vi "CRIO_main.vi"() -> ()   [LabVIEW 2019]
uses:
  <vilib>/Platform/TimedLoop/XDataNode/timing_clust.ctl
  <vilib>/Platform/TimedLoop/XDataNode/nitl_modes.ctl
  <vilib>/Platform/TimedLoop/XDataNode/wakeup.ctl
  <vilib>/DAQmx/read.llb/DAQmx Read (Analog DBL 1Chan 1Samp).vi
  <vilib>/DAQmx/create/channels.llb/DAQmx Create Channel (AI-Voltage-Basic).vi
  <vilib>/DAQmx/configure/timing.llb/DAQmx Timing (Sample Clock).vi
  <vilib>/DAQmx/miscellaneous.llb/DAQmx Fill In Error Info.vi
  <vilib>/platform/TimedLoop/XDataNode/XDataNode.xnode
  <vilib>/Platform/TimedLoop/XDataNode/XDNodeRunTimeDep.lvlib
  <resource>/objmgr/ni.dex.rc
panel:
  out "error out 7":errorcluster
  out "error out 6":errorcluster
  out "Boolean":bool
  out "error out 5":errorcluster
  out "error out 4":errorcluster
  out "error out 3":errorcluster
  out "error out 2":errorcluster
  out "error out":errorcluster
  in  "stop":bool
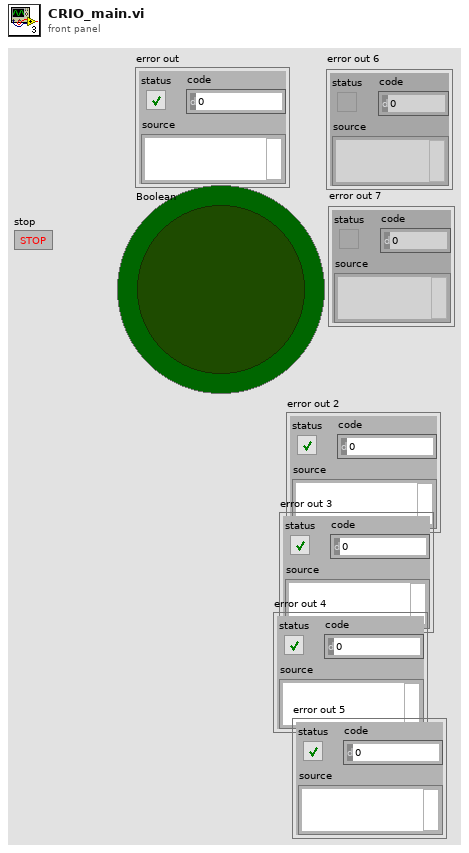
[diagram p1: front panel]
types:
  T1 = typedef "XDNodeRunTimeDep.lvlib/timing_clust.ctl" = cluster{"Expected End [f-1]":u64, "Actual End [f-1]":u64, "Finished Late? [f-1]":bool, "Expected End [i-1]":u64, "Actual End [i-1]":u64, "Finished Late? [i-1]":bool, "Expected Start [i]":u64, "Actual Start [i]":u64, "Expected Start [f]":u64, "Actual Start [f]":u64, "Source Name":string, "Structure Name":string, "Period":i64, "Deadline":i64, "Offset":i64, "Start":i64, "Priority":i32, "Timeout":i32, "Mode":T2, "Wakeup Reason":T3, "Error":errorcluster, "Source Type":string, "Secondary Source Type":string, "Global End Time":u64, "Global Start Time":u64, "Frame Duration":u64, "Iteration Duration":u64, "Assigned CPU":i32, "I/O Scan Engine Mode":u32}
  T2 = typedef "XDNodeRunTimeDep.lvlib/nitl_modes.ctl" = enum32{"No Change", "Process missed periods, maintain original phase", "Discard missed periods, maintain original phase", "Process missed periods, ignore original phase", "Discard missed periods, ignore original phase"}
  T3 = typedef "XDNodeRunTimeDep.lvlib/wakeup.ctl" = enum32{"Normal", "Aborted", "Asynchronous wakeup", "Timing source error", "Timed loop error", "Timeout"}
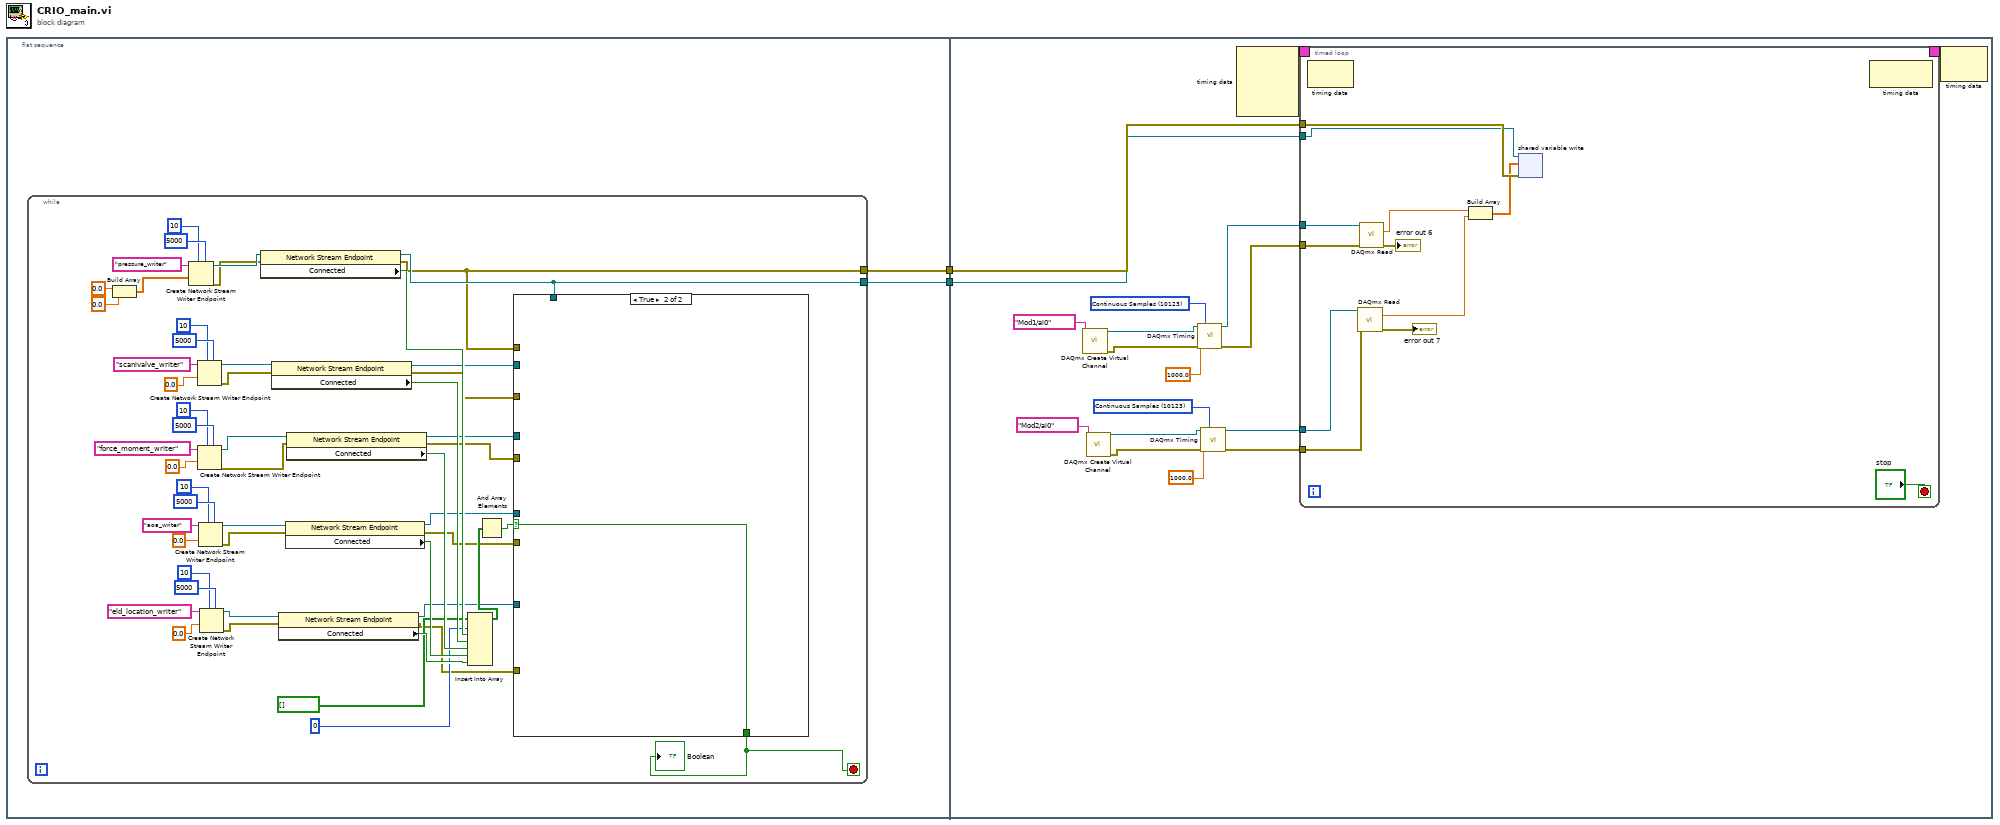
[diagram p0: block diagram]
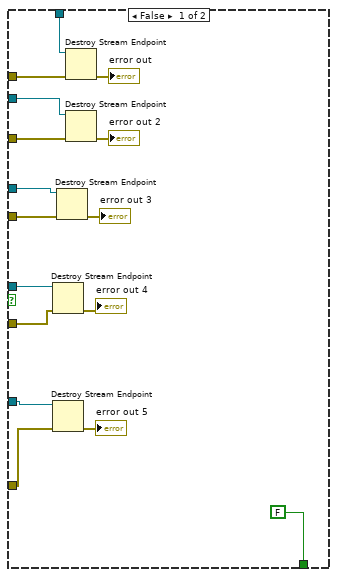
[diagram p2: hidden frame]
diagram:
  n1 = flat-sequence {
    tunnel: [w4] -> w2
    tunnel: [w3] -> w1
    tunnel: w2 -> [w89]
    tunnel: w1 -> [w88]
    frame #0 {
      n2 = while {
        tunnel: [w15] -> w4
        tunnel: [w16] -> w3
        stop <- w8 stop-if-true
        n3 = Build Array(0.0 ("element"), 0.0 ("element")) -> (w5:dbl[])
        n4 = Create Network Stream Writer Endpoint(5:5000 ("timeout in ms (-1)"), 7:10 ("writer buffer size"), 9:w5, 11:"pressure_writer" ("writer name")) -> (0:w36:errorcluster, 3:w37:refnum<k21>)  [unwired: 3 in]
        n5 = Create Network Stream Writer Endpoint(5:5000 ("timeout in ms (-1)"), 7:10 ("writer buffer size"), 9:0.0, 11:"scanivalve_writer" ("writer name")) -> (0:w31:errorcluster, 3:w32:refnum<k21>)  [unwired: 3 in]
        n6 = Create Network Stream Writer Endpoint(5:5000 ("timeout in ms (-1)"), 7:10 ("writer buffer size"), 9:0.0, 11:"force_moment_writer" ("writer name")) -> (0:w29:errorcluster, 3:w30:refnum<k21>)  [unwired: 3 in]
        n7 = Create Network Stream Writer Endpoint(5:5000 ("timeout in ms (-1)"), 7:10 ("writer buffer size"), 9:0.0, 11:"aoa_writer" ("writer name")) -> (0:w25:errorcluster, 3:w26:refnum<k21>)  [unwired: 3 in]
        n8 = Create Network Stream Writer Endpoint(5:5000 ("timeout in ms (-1)"), 7:10 ("writer buffer size"), 9:0.0, 11:"eld_location_writer" ("writer name")) -> (0:w22:errorcluster, 3:w23:refnum<k21>)  [unwired: 3 in]
        n9 = property class="Network Stream Endpoint"(reference=w37, error in=w36) -> (reference out=w16:refnum<k21>, error out=w15:errorcluster, "Connected"=w35:bool)
        n10 = property class="Network Stream Endpoint"(reference=w32, error in=w31) -> (reference out=w18:refnum<k21>, error out=w17:errorcluster, "Connected"=w28:bool)
        n11 = property class="Network Stream Endpoint"(reference=w23, error in=w22) -> (reference out=w10:refnum<k21>, error out=w9:errorcluster, "Connected"=w21:bool)
        n12 = property class="Network Stream Endpoint"(reference=w26, error in=w25) -> (reference out=w12:refnum<k21>, error out=w11:errorcluster, "Connected"=w24:bool)
        n13 = property class="Network Stream Endpoint"(reference=w30, error in=w29) -> (reference out=w14:refnum<k21>, error out=w13:errorcluster, "Connected"=w27:bool)
        n14 = Insert Into Array(array=bool[] [], index=0, new element #1=w35, new element #2=w28, new element #3=w27, new element #4=w24, new element #5=w21) -> (w34:bool[])
        n15 = And Array Elements(Boolean array=w34) -> (logical AND=w33:bool)
        n16 = case shown="True" w33 {
          selector: w33 -> [_ w73]
          tunnel: w18 -> [w67 _]
          tunnel: w17 -> [w66 _]
          tunnel: w16 -> [w65 _]
          tunnel: w15 -> [w64 _]
          tunnel: w14 -> [w63 _]
          tunnel: w13 -> [w62 _]
          tunnel: w12 -> [w61 _]
          tunnel: w11 -> [w60 _]
          tunnel: w10 -> [w59 _]
          tunnel: w9 -> [w58 _]
          tunnel: [FALSE w73] -> w8
          frame False {
            n17 = Destroy Stream Endpoint(8:w60, 11:w61) -> (0:→"error out 4":errorcluster)
            n18 = Destroy Stream Endpoint(8:w58, 11:w59) -> (0:→"error out 5":errorcluster)
            n19 = Destroy Stream Endpoint(8:w62, 11:w63) -> (0:→"error out 3":errorcluster)
            n20 = Destroy Stream Endpoint(8:w64, 11:w65) -> (0:→"error out":errorcluster)
            n21 = Destroy Stream Endpoint(8:w66, 11:w67) -> (0:→"error out 2":errorcluster)
          }
          frame True {
          }
        }
        "Boolean" <- w8
      }
    }
    frame #1 {
      w79 = 10123 items=["Finite Samples"=10178, "Continuous Samples"=10123, "Hardware Timed Single Point"=12522] ("sample mode")
      w86 = 10123 items=["Finite Samples"=10178, "Continuous Samples"=10123, "Hardware Timed Single Point"=12522] ("sample mode")
      n22 = call-poly <vilib>:"DAQmx Create Virtual Channel.vi"("physical channels"=tag "Mod1/ai0") -> ("task out"=w83:refnum<k21>, "error out"=w82:errorcluster)  [unwired: 13 in]
      n23 = call-poly <vilib>:"DAQmx Create Virtual Channel.vi"("physical channels"=tag "Mod2/ai0") -> ("task out"=w77:refnum<k21>, "error out"=w76:errorcluster)  [unwired: 13 in]
      n24 = call-poly <vilib>:"DAQmx Timing.vi"("task/channels in"=w83, "sample mode"=w86, "rate"=1000.0, "error in"=w82) -> ("task out"=w84:refnum<k21>, "error out"=w81:errorcluster)  [unwired: 10 in]
      n25 = call-poly <vilib>:"DAQmx Timing.vi"("task/channels in"=w77, "sample mode"=w79, "rate"=1000.0, "error in"=w76) -> ("task out"=w75:refnum<k21>, "error out"=w74:errorcluster)  [unwired: 10 in]
      n26 = node-c288() -> (w91:T1)  [unwired: 4 in]
      n27 = timed-loop {
        timing: w91 -> [_]
        timing-out: [_] -> w90
        tunnel: w89 -> [w103]
        tunnel: w88 -> [w102]
        tunnel: w84 -> [w100]
        tunnel: w81 -> [w99]
        tunnel: w75 -> [w96]
        tunnel: w74 -> [w95]
        stop <- "stop" stop-if-true
        n28 = node-c288() -> ()  [unwired: 1 in, 1 out]
        n29 = call-poly <vilib>:"DAQmx Read.vi"("task/channels in"=w96, "error in"=w95) -> ("data"=w93:dbl, "error out"=→"error out 7":errorcluster)  [unwired: 11 in, 1 out]
        n30 = call-poly <vilib>:"DAQmx Read.vi"("task/channels in"=w100, "error in"=w99) -> ("data"=w94:dbl, "error out"=→"error out 6":errorcluster)  [unwired: 11 in, 1 out]
        n31 = Build Array(w94, w93) -> (w92:dbl[])
        n32 = shared-variable-write(w102, w103, w92) -> ()  [unwired: 1 in, 3 out]
        n33 = node-c288() -> ()  [unwired: 1 in, 1 out]
      }
      n34 = node-c288(w90) -> ()  [unwired: 1 out]
    }
  }
